vi "Stage2.vi"(8 "Obs Distances Measure Array":dbl[](array[numeric]), 9 "Posture In":dbl[](array[numeric]), 10 "Robot Frame (World)":cluster{"X":sgl, "Y":sgl, "Theta":dbl}, 11 "Start":bool=TRUE) -> (1 "Frame Velocity":dbl[](array[numeric]), 2 "Finish Stage?":bool=TRUE, 3 "Current State":string="Next Goal")   [LabVIEW 2016]
uses:
  MainStateControl.ctl
  WaitVI/Wait Command.ctl
panel:
  out "output cluster":T2
  in  "Init Cluster":T2={"Current State"=enum."Start", "Next Goal"={"X"=0.0, "Y"=0.0, "theta"=0.0}, "Goal Index"=0}
  in  "Goal list":cluster{"X":sgl, "Y":sgl, "theta":dbl}[](array[cluster])=[{"X"=1.5, "Y"=3.48, "theta"=0.0}, {"X"=-0.6, "Y"=3.45, "theta"=-3.12}, {"X"=-0.85, "Y"=-0.12, "theta"=-1.57}, {"X"=5.0, "Y"=5.0, "theta"=0.0}]
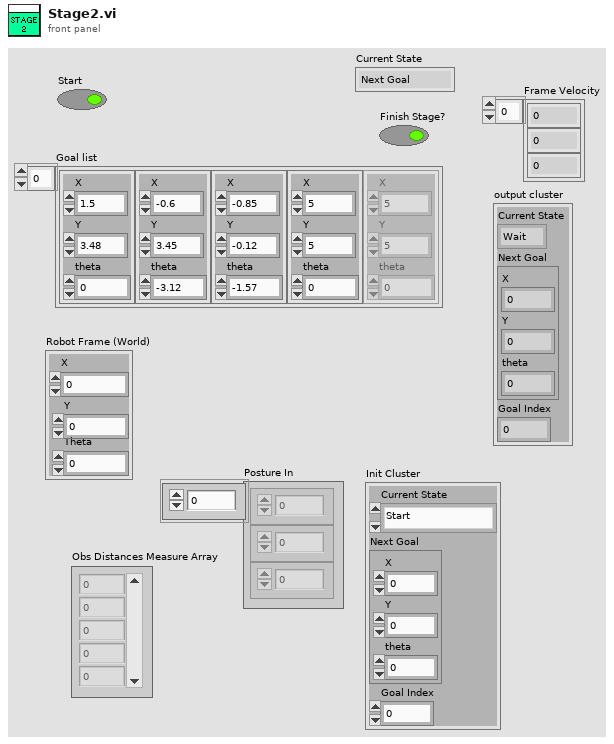
[diagram p1: front panel]
types:
  T1 = typedef "MainStateControl.ctl" = enum16{"Wait", "Next Goal", "Driving", "Start", "Stop"}
  T2 = cluster{"Current State":T1, "Next Goal":cluster{"X":sgl, "Y":sgl, "theta":dbl}, "Goal Index":i32}
  T3 = typedef "Wait Command.ctl" = enum16{"Running", "Init"}
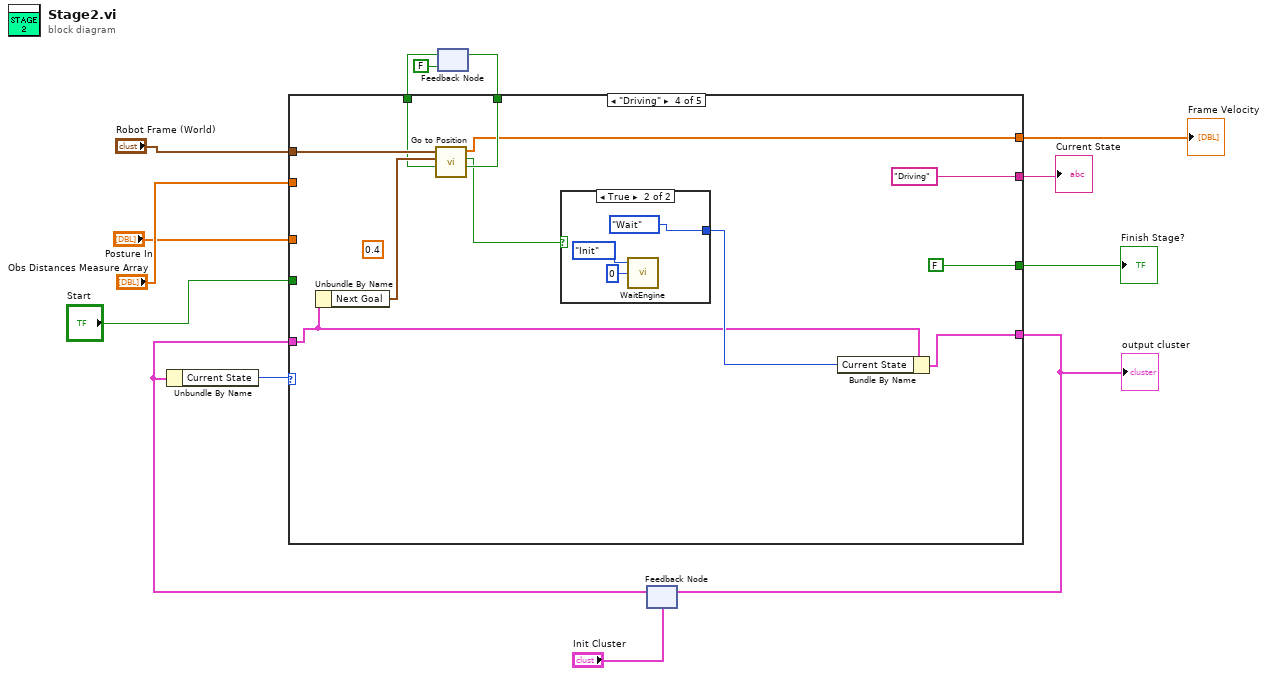
[diagram p0: block diagram]
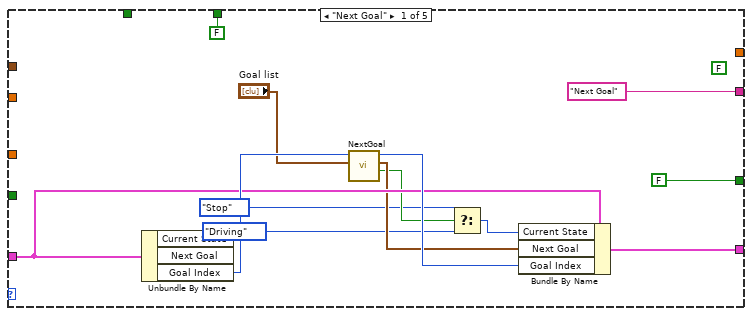
[diagram p2: hidden frame]
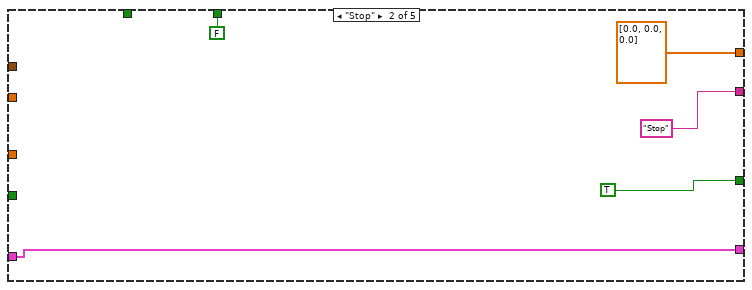
[diagram p3: hidden frame]
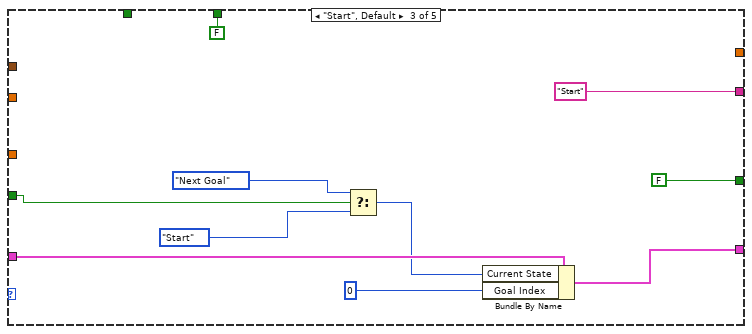
[diagram p4: hidden frame]
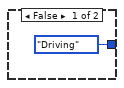
[diagram p5: hidden frame]
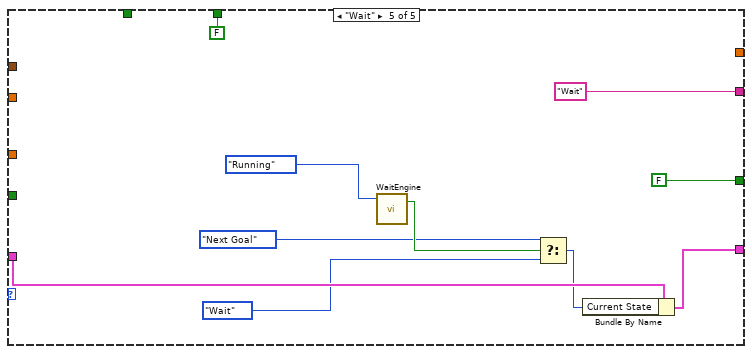
[diagram p6: hidden frame]
diagram:
  n1 = feedback #1(FALSE ("Move Straight Out")) -> (w3:bool)
  n2 = feedback #2("Init Cluster") -> (w10:T2)
  n3 = Unbundle By Name(w10) -> ("Current State"=w11:T1)
  n4 = case shown="\"Driving\"" w11 {
    tunnel: "Start" -> [_ _ w42 _ _]
    tunnel: ["Next Goal" "Stop" "Start" "Driving" "Wait"] -> w13
    tunnel: w10 -> [w24 w32 w39 w49 w65]
    tunnel: [w22 w32 w38 w53 w64] -> w9
    tunnel: [FALSE TRUE FALSE FALSE FALSE] -> w8
    tunnel: "Robot Frame (World)" -> [_ _ _ w48 _]
    tunnel: [_ dbl[] [0.0, 0.0, 0.0] ("Frame Velocity") _ w44 _] -> w6
    tunnel: "Obs Distances Measure Array" -> [_ _ _ _ _]
    tunnel: "Posture In" -> [_ _ _ _ _]
    tunnel: w3 -> [_ _ _ w46 _]
    tunnel: [FALSE ("Move Straight Out") FALSE ("Move Straight Out") FALSE ("Move Straight Out") w45 FALSE ("Move Straight Out")] -> w2
    frame "Next Goal" {
      (unwired) FALSE ("Move Straight Out")
      n5 = Unbundle By Name(w24) -> ("Goal Index"=w26:i32)  [unwired: 2 out]
      n6 = call "NextGoal.vi"("Goal list"="Goal list", "Current Index"=w26) -> ("Finish track?"=w21:bool, "Next Goal"=w23:cluster{"X":sgl, "Y":sgl, "theta":dbl}, "Goal Index"=w25:i32)  [unwired: 7 in]
      n7 = Select(t=MainStateControl."Stop" ("Enum"), s=w21, f=MainStateControl."Driving" ("Enum")) -> (s? t:f=w19:T1)
      n8 = Bundle By Name(cluster=w24, "Current State"=w19, "Next Goal"=w23, "Goal Index"=w25) -> (w22:T2)
    }
    frame "Stop" {
    }
    frame "Start", Default {
      n9 = Select(t=MainStateControl."Next Goal", s=w42, f=MainStateControl."Start") -> (s? t:f=w37:T1)
      n10 = Bundle By Name(cluster=w39, "Current State"=w37, "Goal Index"=0) -> (w38:T2)
    }
    frame "Driving" {
      (unwired) 0.4 ("V Forward")
      n11 = Unbundle By Name(w49) -> ("Next Goal"=w47:cluster{"X":sgl, "Y":sgl, "theta":dbl})
      n12 = call "Go to Position.vi"("Move Straight In"=w46, "Goal Frame (World)"=w47, "Robot Frame (World)"=w48) -> ("Move Straight Out"=w45:bool, "Goal Arrive?"=w43:bool, "Frame Velocity"=w44:dbl[])  [unwired: 6 in]
      n13 = case shown="True" w43 {
        tunnel: [MainStateControl."Driving" ("Enum") MainStateControl."Wait" ("Enum")] -> w51
        frame False {
        }
        frame True {
          n14 = call "WaitEngine.vi"("Wait Time (ms)"=u32 0, "Wait Command"=Wait_Command."Init") -> ()  [unwired: 2 in, 1 out]
        }
      }
      n15 = Bundle By Name(cluster=w49, "Current State"=w51) -> (w53:T2)
    }
    frame "Wait" {
      n16 = call "WaitEngine.vi"("Wait Command"=Wait_Command."Running") -> ("Elapsed?"=w66:bool)  [unwired: 3 in]
      n17 = Select(t=MainStateControl."Next Goal" ("Enum"), s=w66, f=MainStateControl."Wait" ("Enum")) -> (s? t:f=w62:T1)
      n18 = Bundle By Name(cluster=w65, "Current State"=w62) -> (w64:T2)
    }
  }
  "Current State" <- w13
  "output cluster" <- w9
  "Finish Stage?" <- w8
  "Frame Velocity" <- w6
  n19 = feedback-in #1(w2) -> ()
  n20 = feedback-in #2(w9) -> ()
